vi "full pattern analyze+remembering (SubVI).vi"(8 "error in (no error)":errorcluster, 9 "divider":sgl=1.6, 10 "Angle (degrees)":sgl, 11 "Patterns to remember":i32=3) -> (0 "error out":errorcluster, 2 "Pattern classes out":i32[](array[numeric]), 3 "Pattern":i32)   [LabVIEW 2017]
uses:
  <vilib>/vision/Pattern Matching.llb/IMAQ GM Match Report.ctl
  <vilib>/userdefined/High Color/IMAQdx.ctl
  <vilib>/myRIO/Instrument Drivers/Onboard IO/DIO/typedefs/DIO Reference.ctl
  <vilib>/myRIO/Common/Instrument Driver Framework/Utilities/typedefs/myRIO Generic Hardware Reference.ctl
  <vilib>/myRIO/Common/Instrument Driver Framework/Utilities/typedefs/Hardware Version Enum.ctl
  <vilib>/myRIO/Common/Instrument Driver Framework/Utilities/typedefs/myRIO v1.0 Reference.ctl
  <vilib>/myRIO/Common/Instrument Driver Framework/Utilities/typedefs/Generic FPGA Reference.ctl
  <vilib>/myRIO/Common/Instrument Driver Framework/myRIO v1.0/DIO/typedefs/DIO Channels List.ctl
  <vilib>/myRIO/Common/Instrument Driver Framework/myRIO v1.0/DIO/typedefs/DIO Channels Enum.ctl
  <vilib>/userdefined/High Color/nirio_resource_hc.ctl
  <vilib>/myRIO/Common/Instrument Driver Framework/Utilities/vis/Is FPGA Ref Available.vi
  <vilib>/myRIO/Common/Instrument Driver Framework/myRIO v1.0/DIO/vis/myRIO v1.1 Open DIO.vi
  <vilib>/myRIO/Instrument Drivers/Onboard IO/DIO/vis/Read.vi
  <vilib>/myRIO/Common/Instrument Driver Framework/Utilities/vis/Validate Channels.vi
  <vilib>/myRIO/Common/Instrument Driver Framework/myRIO v1.0/DIO/vis/myRIO v1.0 Reserve DIO.vi
  <vilib>/myRIO/Common/Instrument Driver Framework/myRIO v1.0/Resource Manager/vis/myRIO v1.0 Reserve Channel List.vi
  <vilib>/myRIO/Common/Instrument Driver Framework/myRIO v1.0/DIO/vis/myRIO v1.0 Build MUX Configuration DIO.vi
  <vilib>/myRIO/Common/Instrument Driver Framework/myRIO v1.0/Resource Manager/vis/myRIO v1.0 Reserve Channel.vi
  <vilib>/myRIO/Common/Instrument Driver Framework/myRIO v1.0/Resource Manager/vis/myRIO v1.0 Unreserve Channel.vi
  <vilib>/myRIO/Common/Instrument Driver Framework/myRIO v1.0/Resource Manager/vis/myRIO v1.0 Create Configuration List.vi
  <vilib>/myRIO/Common/Instrument Driver Framework/myRIO v1.0/Resource Manager/vis/myRIO v1.0 Build Mutex Name.vi
  <vilib>/Utility/VariantDataType/GetNumericInfo.vi
  <vilib>/Utility/error.llb/Error Cluster From Error Code.vi
  <vilib>/myRIO/Common/Instrument Driver Framework/myRIO v1.0/myRIO v1.1 Open.vi
  <vilib>/myRIO/Common/Instrument Driver Framework/Utilities/vis/IO Manager.vi
  <vilib>/myRIO/Common/Instrument Driver Framework/Utilities/vis/Configuration Manager.vi
  <vilib>/myRIO/Common/Instrument Driver Framework/myRIO v1.0/Resource Manager/vis/myRIO v1.0 Configure IO.vi
  <vilib>/myRIO/Common/Instrument Driver Framework/myRIO v1.0/myRIO v1.0 Close.vi
  <vilib>/myRIO/Common/Instrument Driver Framework/myRIO v1.0/DIO/vis/myRIO v1.0 Read DIO.vi
  <vilib>/myRIO/Express VI/Onboard Devices/Button/Button Express VI.xnode
  <vilib>/myRIO/Instrument Drivers/Onboard IO/DIO/vis/myRIO DIO Open.xnode
  <vilib>/vision/NI_Vision_Development_Module.lvlib
  <vilib>/vision/driver/NI_Vision_Acquisition_Software.lvlib
  <vilib>/myRIO/Instrument Drivers/Onboard IO/DIO/DIO.lvlib
panel:
  in  "Start":bool
  in  "Stop Button":bool
  out "CurPattern":i32
  in  "Continue":bool
  in  "Pattern classes":i32[](array[numeric])
  out "x0":i32
  out "Scale":sgl
  out "y0":i32
  out "x1":i32
  out "y1":i32
  in  "ROI":T1={"Global Rectangle"=[109, 72, 345, 284], "Contours"=[{"ID"=enum."External", "Type"=3, "Coordinates"=[109, 72, 345, 284]}]} {"Contours"."Type" items=["No Selection", "Point", "Line", "Rectangle", "Oval", "Polygon", "Freehand Region", "Annulus", "Unused2", "Unused3", "Broken Line", "Freehand Line", "Rotated Rectangle"]}
  out "Number of Matches":i32
  out "Calibrated Matches":T2[](array[typedef]) {"Correlation Score" format="%.2f"; "Target Template Curve Score" format="%.2f"; "Template Target Curve Score" format="%.2f"; "Bounding Box"."y" format="%.2f"; "Bounding Box"."x" format="%.2f"; "Position"."y" format="%.2f"; "Position"."x" format="%.2f"; "Score" format="%.2f"; "Scale" format="%.2f"; "Angle" format="%.2f"; "Occlusion %" format="%.2f"}
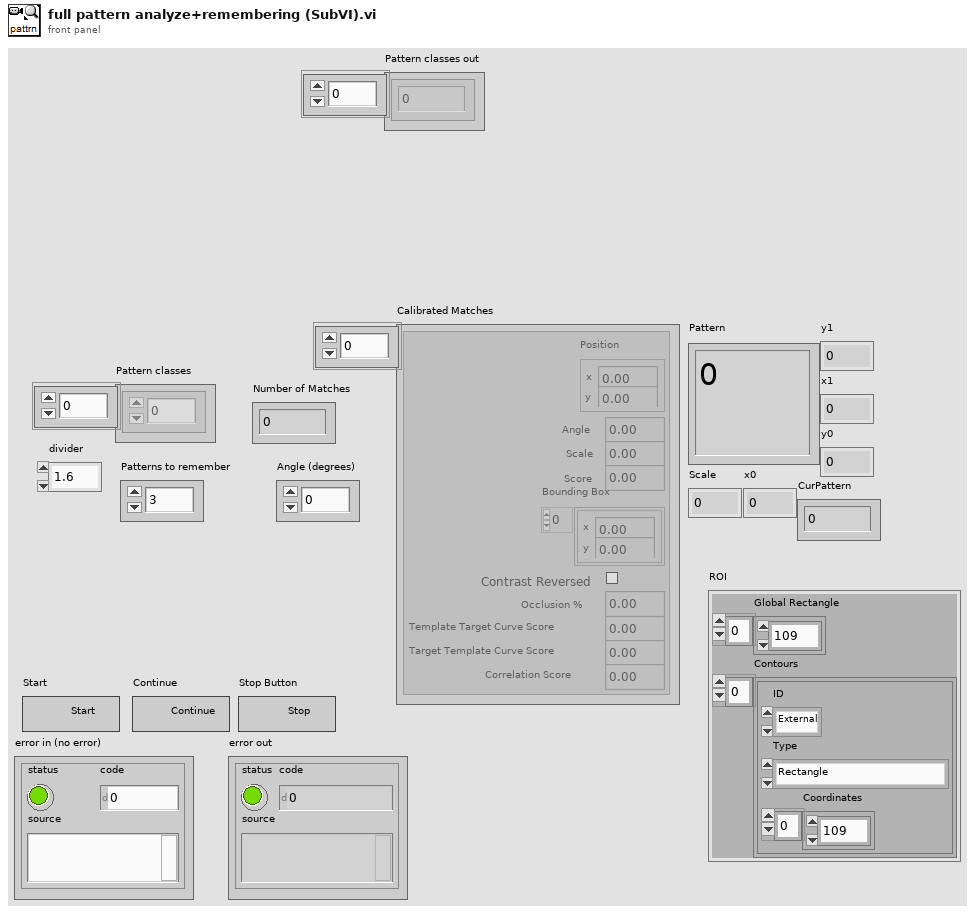
[diagram p1: front panel]
types:
  T1 = cluster{"Global Rectangle":i32[], "Contours":cluster{"ID":enum32{"External", "Internal"}, "Type":u32, "Coordinates":i32[]}[]}
  T2 = typedef "IMAQ GM Match Report.ctl" = cluster{"Position":cluster{"x":sgl, "y":sgl}, "Angle":sgl, "Scale":sgl, "Score":sgl, "Bounding Box":cluster{"x":sgl, "y":sgl}[], "Contrast Reversed":bool, "Occlusion %":sgl, "Template Target Curve Score":sgl, "Target Template Curve Score":sgl, "Correlation Score":sgl}
  T3 = typedef "IMAQdx.ctl" = refnum<k21>
  T4 = typedef "DIO.lvlib/DIO Reference.ctl" = cluster{"myRIO Reference":T5, "DIO Channels List":T9}
  T5 = typedef "myRIO Generic Hardware Reference.ctl" = cluster{"myRIO Model":T6, "myRIO Hardware Reference":T7}
  T6 = typedef "Hardware Version Enum.ctl" = enum16{"Unknown", "myRIO-1900", "myRIO-1950", "roboRIO", "NI ELVIS RIO CM"}
  T7 = typedef "myRIO v1.0 Reference.ctl" = cluster{"Generic FPGA Reference":T8, "Allow multiple opens":bool}
  T8 = typedef "Generic FPGA Reference.ctl" = refnum<k20>
  T9 = typedef "DIO Channels List.ctl" = T10[]
  T10 = typedef "DIO Channels Enum.ctl" = enum16{"Not Connected", "C/DIO0", "C/DIO1", "C/DIO2", "C/DIO3", "C/DIO4", "C/DIO5", "C/DIO6", "C/DIO7", "A/DIO0", "A/DIO1", "A/DIO2", "A/DIO3", "A/DIO4", "A/DIO5", "A/DIO6", "A/DIO7", "A/DIO8", "A/DIO9", "A/DIO10", "A/DIO11", "A/DIO12", "A/DIO13", "A/DIO14", "A/DIO15", "B/DIO0", "B/DIO1", "B/DIO2", "B/DIO3", "B/DIO4", "B/DIO5", "B/DIO6", "B/DIO7", "B/DIO8", "B/DIO9", "B/DIO10", "B/DIO11", "B/DIO12", "B/DIO13", "B/DIO14", "B/DIO15", "LED0", "LED1", "LED2", "LED3", "Button0", "DIO/DIO0", "DIO/DIO1", "DIO/DIO2", "DIO/DIO3", "DIO/DIO4", "DIO/DIO5", "DIO/DIO6", "DIO/DIO7", "DIO/DIO8", "DIO/DIO9", "SPI/CS0", "SPI/CS1", "SPI/CS2", "SPI/CS3", "LED RADIO (Green)", "LED RADIO (Red)", "LED COMM (Green)", "LED COMM (Red)", "LED MODE (Green)", "LED MODE (Red)"}
  T11 = typedef "nirio_resource_hc.ctl" = tag
  T12 = typedef "IMAQ Image.ctl" = refnum<image>
  T13 = cluster{"ID":enum32{"External", "Internal"}, "Type":u32, "Coordinates":i32[]}[]
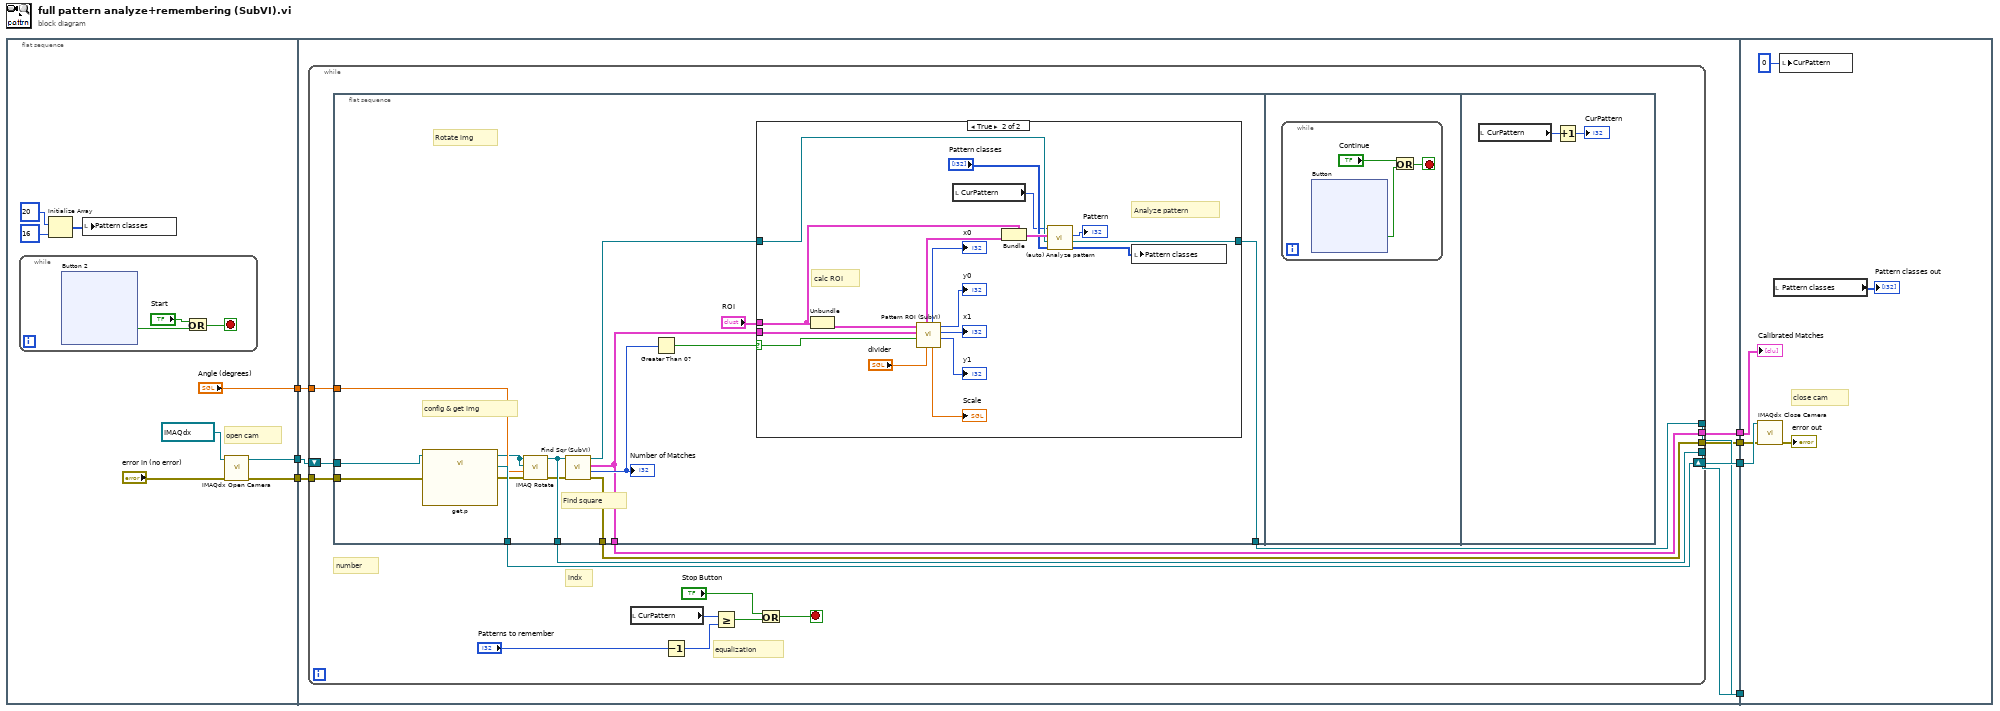
[diagram p0: block diagram]
diagram:
  n1 = flat-sequence {
    tunnel: [w12] -> w8
    tunnel: [w9] -> w7
    tunnel: ["Angle (degrees)"] -> w6
    tunnel: w8 -> [w61]
    tunnel: w7 -> [w60]
    tunnel: w6 -> [w59]
    tunnel: [w62] -> w5
    tunnel: [w58] -> w4
    tunnel: [w57] -> w3
    tunnel: [w56] -> w2
    tunnel: [w55] -> w1
    tunnel: w5 -> [w154]
    tunnel: w4 -> [_]
    tunnel: w3 -> [w155]
    tunnel: w2 -> [_]
    tunnel: w1 -> [w153]
    frame #0 {
      # "open cam"
      n2 = while {
        stop <- w18 stop-if-true
        n3 = xnode "Button 2"() -> ("Value"=w17:bool)  [unwired: 1 in, 1 out]
        n4 = Or(x="Start", y=w17) -> (x .or. y?=w18:bool)
      }
      n5 = Initialize Array(20 ("element"), 16 ("dimension size")) -> (w16:i32[])
      n6 = local write "Pattern classes"(w16) -> ()
      n7 = call <vilib>:"IMAQdx Open Camera.vi"("error in"="error in (no error)", "Session In"=T3 "cam0") -> ("error out"=w9:errorcluster, "Session Out"=w12:T3)  [unwired: 8 in]
    }
    frame #1 {
      n8 = while {
        tunnel: w60 -> [w74]
        tunnel: w59 -> [w73]
        tunnel: [w72] -> w58
        tunnel: [w71] -> w57
        tunnel: [w70] -> w56
        shift-right: [w76] -> w62
        shift-left: w61 -> [w75]
        tunnel: [w69] -> w55
        stop <- w68 stop-if-true
        # "equalization"
        # "number"
        # "indx"
        n9 = flat-sequence {
          tunnel: [w91] -> w76
          tunnel: w75 -> [w90]
          tunnel: w74 -> [w89]
          tunnel: w73 -> [w87]
          tunnel: [w85] -> w72
          tunnel: [w80] -> w71
          tunnel: [w78] -> w70
          tunnel: [w77] -> w69
          frame #0 {
            # "config & get img"
            # "Rotate img"
            # "Find square"
            n10 = call "get.p.vi"("Session in"=w90, "error in"=w89) -> ("Image Out"=w86:T12, "Session Out"=w91:T3, "error out"=w88:errorcluster)  [unwired: 23 in]
            n11 = call "IMAQ Rotate"("error in (no error)"=w88, "Angle (degrees)"=w87, "Image Dst"=w86, "Image Src"=w86) -> ("error out"=w84:errorcluster, "Image Dst Out"=w85:T12)  [unwired: 6 in]
            n12 = call "Find Sqr (SubVI).vi"("error in (no error)"=w84, "Refnum in"=w85) -> ("error out"=w77:errorcluster, "Number of Matches (Geometric Matching 1)"=w83:i32, "Calibrated Matches (Geometric Matching 1)"=w80:T2[], "Refnum out"=w79:T12)  [unwired: 6 in]
            "Number of Matches" <- w83
            n13 = Greater Than 0?(x=w83) -> (x > 0?=w82:bool)
            n14 = case shown="True" w82 {
              selector: w82 -> [_ w108]
              tunnel: "ROI" -> [_ w107]
              tunnel: w80 -> [_ w109]
              tunnel: w79 -> [w92 w104]
              tunnel: [w92 w103] -> w78
              frame False {
              }
              frame True {
                # "Analyze pattern"
                # "calc ROI"
                n15 = Unbundle(w107) -> ("Contours"=w110:T13)  [unwired: 1 out]
                n16 = call "Pattern ROI (SubVI).vi"("divider"="divider", "number of matches"=w108, "Calibrated Matches (Geometric Matching 1)"=w109, "Contours in"=w110) -> ("y1"=→"y1":i32, "x1"=→"x1":i32, "y0"=→"y0":i32, "Scale"=→"Scale":sgl, "x0"=→"x0":i32, "Contours out"=w106:T13)  [unwired: 2 in]
                n17 = local read "CurPattern"() -> (w94:i32)
                n18 = Bundle(cluster=w107, "Contours"=w106) -> (w105:T1)  [unwired: 1 in]
                n19 = call "(auto) Analyze pattern.vi"("Pattern classes"="Pattern classes", "Image In"=w104, "ROI Descriptor (Image Mask 1)"=w105, "pattern number"=w94) -> ("output array"=w93:i32[], "Image Out"=w103:T12, "Pattern"=→"Pattern":i32)  [unwired: 5 in]
                n20 = local write "Pattern classes"(w93) -> ()
              }
            }
          }
          frame #1 {
            n21 = while {
              stop <- w112 stop-if-true
              n22 = xnode "Button"() -> ("Value"=w111:bool)  [unwired: 1 in, 1 out]
              n23 = Or(x="Continue", y=w111) -> (x .or. y?=w112:bool)
            }
          }
          frame #2 {
            n24 = local read "CurPattern"() -> (w149:i32)
            n25 = Increment(x=w149) -> (x+1=→"CurPattern":i32)
          }
        }
        n26 = local read "CurPattern"() -> (w64:i32)
        n27 = Decrement(x="Patterns to remember") -> (x-1=w63:i32)
        n28 = Greater Or Equal?(x=w64, y=w63) -> (x >= y?=w66:bool)
        n29 = Or(x="Stop Button", y=w66) -> (x .or. y?=w68:bool)
      }
    }
    frame #2 {
      # "close cam"
      n30 = call <vilib>:"IMAQdx Close Camera.vi"("error in"=w153, "Session In"=w154) -> ("error out"=→"error out":errorcluster)  [unwired: 9 in]
      n31 = local read "Pattern classes"() -> (→"Pattern classes out":i32[])
      n32 = local write "CurPattern"(0 ("CurPattern")) -> ()
      "Calibrated Matches" <- w155
    }
  }
